vi "Test register Click event.vi"(11 "Test Case In":refnum<class "Test Cases.lvclass">) -> (0 "error out":errorcluster, 3 "Test Case Out":refnum<class "Test Cases.lvclass">)   [LabVIEW 2024, in "Test Cases.lvclass"]
uses:
  Test Cases.lvclass
  C:/Program Files/National Instruments/LabVIEW 2024/vi.lib/Astemes/LUnit/Test Case.lvclass
  <vilib>/Utility/Data Type/Type Definitions/Data Type.ctl
  MyEventGrid/MyEventGrid.lvclass
  D:/git/Sourcegrid-LabVIEW/source/Grid/SourceGrid.lvclass
  MyEventGrid/MyEventGrid.lvclass/MyEventGrid.ctl
  <vilib>/Astemes/LUnit/Test Case.lvclass/Test Case.ctl
  <vilib>/Astemes/LUnit/Append Pass Result.vi
  <vilib>/Astemes/LUnit/Append Fail Result.vi
  <vilib>/Astemes/LUnit/Run In UI.vi
  <vilib>/Utility/error.llb/Clear Errors.vi
  <vilib>/Astemes/LUnit/Test Case.lvclass
  source/Grid/SourceGrid.lvclass
  source/Cells/Cell Context/Cell Context.lvclass
  <vilib>/Utility/Data Type/NI_Data Type.lvlib
  D:/git/Sourcegrid-LabVIEW/dll/SourceGrid.dll
  dll/SourceGrid.dll
panel:
  in  "stop":bool
  out "onValueChanged Value":variant
  out "onValueChanged Value type":T1
  out "onClick Position":string
  out "onClick Value":variant
  in  "Grid Container":refnum<k24>(container)
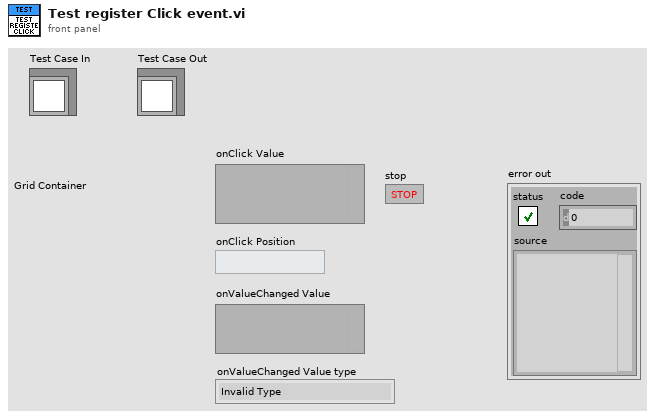
[diagram p1: front panel]
types:
  T1 = typedef "NI_Data Type.lvlib/Data Type.ctl" = enum8{"Invalid Type", "Void", "I8", "I16", "I32", "I64", "U8", "U16", "U32", "U64", "Single Float", "Double Float", "Extended Float", "Single Complex", "Double Complex", "Extended Complex", "Enum U8", "Enum U16", "Enum U32", "Enum U64", "Single Float With Unit", "Double Float With Unit", "Extended Float With Unit", "Single Complex with Unit", "Double Complex with Unit", "Extended Complex with Unit", "Boolean", "String", "Path", "Picture", "Tag", "Array", "Cluster", "Variant", "LV Variant", "Waveform", "Timestamp", "Digital Waveform", "Digital Data", "ExpressData", "Refnum", "External Data", "VI", "Poly VI", "LabVIEW Class Instance", "Fixed Point", "Set Collection", "Map Collection"}
  T2 = cluster{"onClick":refnum<user-event>, "onDoubleClick":refnum<user-event>, "onValueChanged":refnum<user-event>}
  T3 = typedef "Rendezvous RefNum" = refnum<k1>
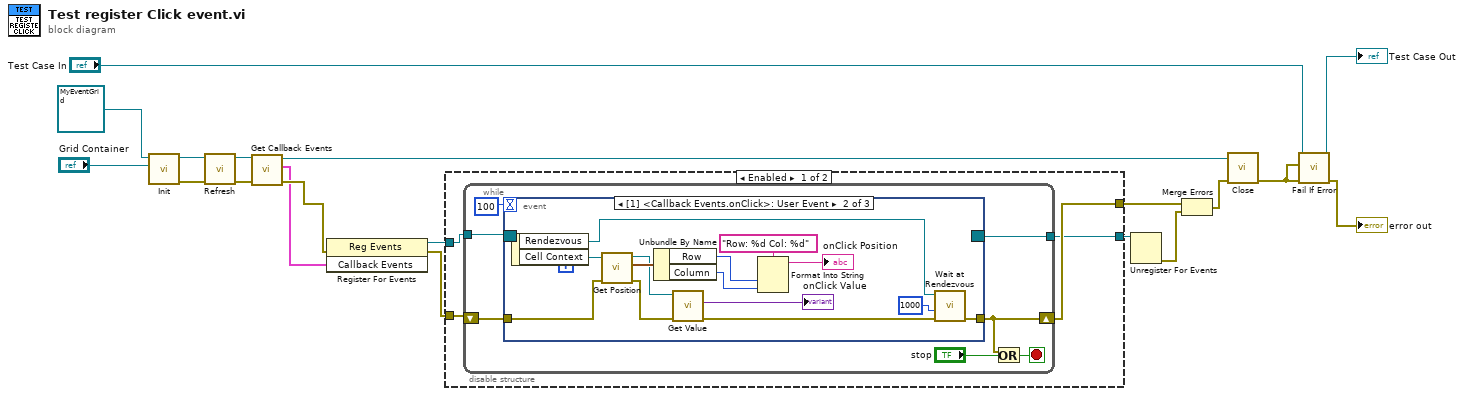
[diagram p0: block diagram]
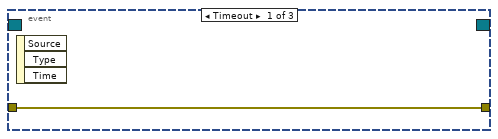
[diagram p2: hidden frame]
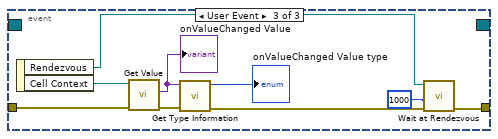
[diagram p3: hidden frame]
diagram:
  n1 = call-dynamic "Init.vi"("Sourcegrid Container"="Grid Container", "MyEventGrid in"=refnum<class "MyEventGrid.lvclass"> refnum ("Grid in")) -> ("error out"=w12:errorcluster, "MyEventGrid out"=w11:refnum<class "MyEventGrid.lvclass">)  [unwired: 8 in]
  n2 = call "Refresh.vi"("error in"=w12, "SourceGrid in"=w11) -> ("error out"=w13:errorcluster, "SourceGrid out"=w10:refnum<class "MyEventGrid.lvclass">)  [unwired: 8 in]
  n3 = call "Get Callback Events.vi"("MyEventGrid in"=w10) -> ("Callback Events"=w7:T2, "MyEventGrid out"=w9:refnum<class "MyEventGrid.lvclass">)  [unwired: 9 in]
  n4 = register-events(error in=w13, w7) -> (reference out=w5:refnum<event-registration>, error out=w4:errorcluster)  [unwired: 1 in]
  n5 = disable-structure shown="Enabled" {
    disable-tunnel: [w20 w55] -> w6
    disable-tunnel: w5 -> [w19 w55]
    disable-tunnel: w4 -> [w22 w54]
    disable-tunnel: [w21 w54] -> w1
    frame Enabled {
      n6 = while {
        tunnel: w19 -> [w28]
        tunnel: [w27] -> w20
        shift-right: [w24] -> w21
        shift-left: w22 -> [w23]
        stop <- w25 stop-if-true
        n7 = event shown="[1] <Callback Events.onClick>: User Event" {
          selector: w28 -> [_ _ _]
          dyn-events: [_ _ _] -> w27
          timeout: 100 -> [_ _ _]
          tunnel: [w30 w34 w45] -> w24
          tunnel: w23 -> [w30 w37 w52]
          event Timeout {
            n8 = event-data() -> ()  [unwired: 1 in, 3 out]
          }
          event User Event {
            n9 = event-data() -> ("Rendezvous"=w33:T3, "Cell Context"=w44:refnum<class "Cell Context.lvclass">)  [unwired: 1 in]
            n10 = call "Get Position.vi"("error in"=w37, "Cell Context in"=w44) -> ("error out"=w38:errorcluster, "Position"=w43:cluster{"Row":i32, "Column":i32}, "Cell Context out"=w36:refnum<class "Cell Context.lvclass">)  [unwired: 7 in]
            n11 = Unbundle By Name(w43) -> ("Row"=w40:i32, "Column"=w39:i32)
            n12 = call "Get Value.vi"("error in (no error)"=w38, "Cell Context in"=w36) -> ("error out"=w32:errorcluster, "Value"=→"onClick Value":variant)  [unwired: 7 in, 1 out]
            n13 = Format Into String(format string="Row: %d Col: %d", w40, w39) -> (resulting string=→"onClick Position":string)  [unwired: 2 in, 1 out]
            n14 = call <vilib>:"Wait at Rendezvous.vi"("error in (no error)"=w32, "ms timeout (-1)"=1000, "rendezvous"=w33) -> ("error out"=w34:errorcluster)  [unwired: 2 in, 2 out]
          }
          event User Event {
            n15 = event-data() -> ("Rendezvous"=w48:T3, "Cell Context"=w53:refnum<class "Cell Context.lvclass">)  [unwired: 1 in]
            n16 = call "Get Value.vi"("error in (no error)"=w52, "Cell Context in"=w53) -> ("error out"=w50:errorcluster, "Value"=w51:variant)  [unwired: 7 in, 1 out]
            "onValueChanged Value" <- w51
            n17 = call <vilib>:"Get Type Information.vi"("error in (no error)"=w50, "variant"=w51) -> ("error out"=w47:errorcluster, "type"=→"onValueChanged Value type":T1)  [unwired: 5 in, 3 out]
            n18 = call <vilib>:"Wait at Rendezvous.vi"("error in (no error)"=w47, "ms timeout (-1)"=1000, "rendezvous"=w48) -> ("error out"=w45:errorcluster)  [unwired: 2 in, 2 out]
          }
        }
        n19 = Or(x=w24, y="stop") -> (x .or. y?=w25:bool)
      }
    }
    frame Disabled {
    }
  }
  n20 = Unregister For Events(event registration refnum=w6) -> (error out=w2:errorcluster)  [unwired: 1 in]
  n21 = Merge Errors(w1, w2) -> (w3:errorcluster)
  n22 = call-dynamic "Close.vi"("error in"=w3, "MyEventGrid in"=w9) -> ("error out"=w8:errorcluster)  [unwired: 8 in, 1 out]
  n23 = call <vilib>:"Fail If Error.vi"("error in (no error)"=w8, "Assert error"=w8, "LUnit Test Case In"="Test Case In") -> ("error out"=→"error out":errorcluster, "LUnit Test Case Out"=→"Test Case Out":refnum<class "Test Cases.lvclass">)  [unwired: 7 in]
